vi "Check for Cancel.vi"(8 "error in":errorcluster, 11 "Peer Review in":refnum<class "Peer Review.lvclass">) -> (0 "error out":errorcluster, 3 "Peer Review out":refnum<class "Peer Review.lvclass">)   [LabVIEW 2020, in "Peer Review.lvclass"]
uses:
  Peer Review.lvclass
  Peer Review.lvclass/Peer Review.ctl
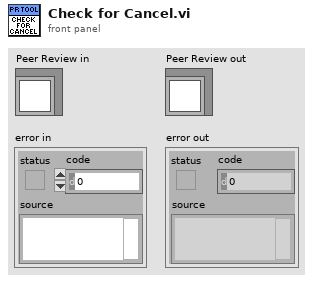
[diagram p1: front panel]
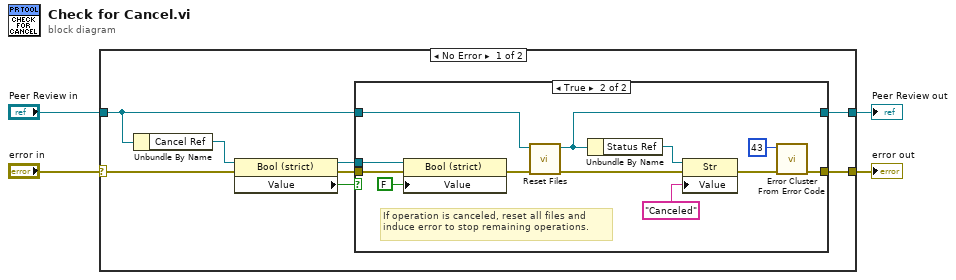
[diagram p0: block diagram]
diagram:
  n1 = case shown="No Error" "error in" {
    selector: "error in" -> [w11 w28]
    tunnel: [w7 w28] -> w3
    tunnel: "Peer Review in" -> [w6 w27]
    tunnel: [w5 w27] -> w1
    frame No Error {
      n2 = Unbundle By Name(w6) -> ("Cancel Ref"=w12:refnum<vi>)
      n3 = property class="Bool (strict)"(reference=w12, error in=w11) -> (reference out=w8:refnum<vi>, error out=w9:errorcluster, "Value"=w10:bool)
      n4 = case shown="True" w10 {
        tunnel: w9 -> [w14 w24]
        tunnel: w8 -> [_ w26]
        tunnel: [w14 w22] -> w7
        tunnel: w6 -> [w13 w20]
        tunnel: [w13 w16] -> w5
        frame False {
        }
        frame True {
          # "If operation is canceled, reset all files and induce error to stop remaining operations."
          n5 = property class="Bool (strict)"(reference=w26, error in=w24, "Value"=FALSE) -> (error out=w21:errorcluster)  [unwired: 1 out]
          n6 = call "Reset Files.vi"("error in"=w21, "Peer Review in"=w20) -> ("error out"=w18:errorcluster, "Peer Review out"=w16:refnum<class "Peer Review.lvclass">)  [unwired: 8 in]
          n7 = Unbundle By Name(w16) -> ("Status Ref"=w15:refnum<vi>)
          n8 = property on="Property Node" class="Str"(reference=w15, error in=w18, "Value"="Canceled") -> (error out=w17:errorcluster)  [unwired: 1 out]
          n9 = call <vilib>:"Error Cluster From Error Code.vi"("error in (no error)"=w17, "error code (0)"=43) -> ("error out"=w22:errorcluster)  [unwired: 7 in]
        }
      }
    }
    frame Error {
    }
  }
  "error out" <- w3
  "Peer Review out" <- w1
